vi "PSTR-Check If Repair Needed.vi"(0 "Data in":T2, 9 "CFTS-PSTR":T1) -> (8 "needs repair":bool)   [LabVIEW 2020]
uses:
  Typedefs/PSTR-Data.ctl
  Typedefs/PSTR-Model Fit.ctl
  Typedefs/PSTR-Fit Parameters.ctl
  Typedefs/PSTR-File Info.ctl
  <vilib>/Analysis/baseanly.llb/Mean (DBL).vi
  <vilib>/Analysis/NI_AALBase.lvlib
  <vilib>/Analysis/NI_AALPro.lvlib
panel:
  # "NF x NL x 2 x Npts"
  # "NF x NL x Npts"
  # "NF x NL"
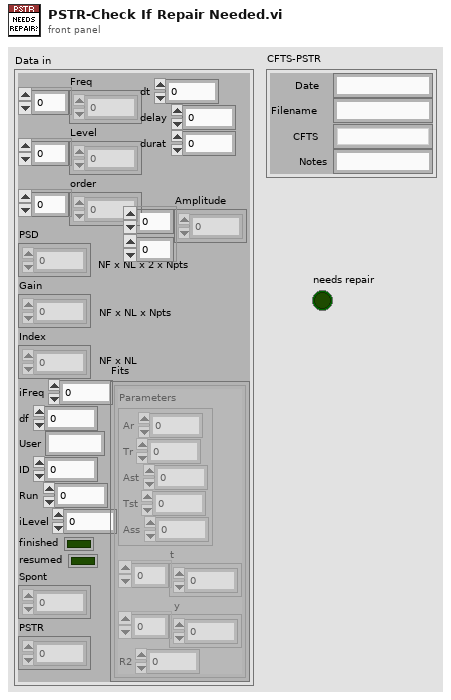
[diagram p1: front panel]
types:
  T1 = typedef "PSTR-File Info.ctl" = cluster{"Date":string, "Filename":string, "CFTS":string, "Notes":string}
  T2 = typedef "PSTR-Data.ctl" = cluster{"Freq":dbl[], "Level":dbl[], "order":i32[], "PSD":dbl[][][][], "Gain":dbl[][][], "Index":dbl[][], "iFreq":i32, "df":dbl, "User":string, "ID":i32, "Run":i32, "iLevel":i32, "finished":bool, "resumed":bool, "Spont":dbl[][], "PSTR":dbl[][][], "dt":dbl, "delay":dbl, "durat":dbl, "Fits":T3[][], "Amplitude":dbl[][]}
  T3 = typedef "PSTR-Model Fit.ctl" = cluster{"Parameters":T4, "t":dbl[], "y":dbl[], "R2":dbl}
  T4 = typedef "PSTR-Fit Parameters.ctl" = cluster{"Ar":dbl, "Tr":dbl, "Ast":dbl, "Tst":dbl, "Ass":dbl}
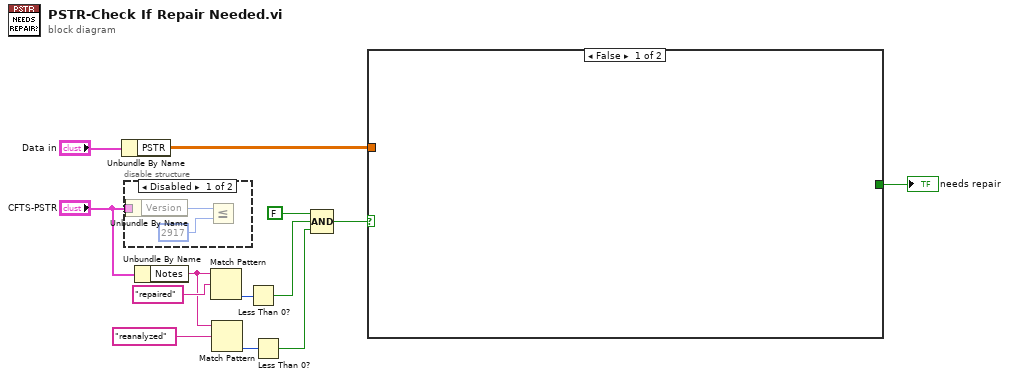
[diagram p0: block diagram]
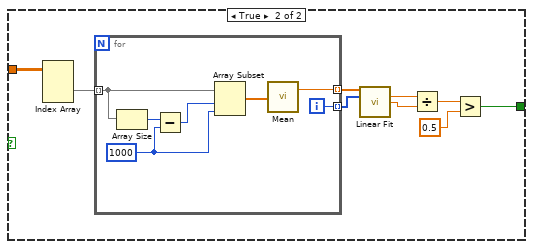
[diagram p3: hidden frame]
diagram:
  n1 = Unbundle By Name("Data in") -> ("PSTR"=w4:dbl[][][])
  n2 = disable-structure shown="Disabled" {
    disable-tunnel: "CFTS-PSTR" -> [w14 _]
    frame Disabled {
      n3 = Unbundle By Name(w14) -> ("Version"=w16:i32)
      n4 = Less Or Equal?(x=w16, y=2917) -> ()  [unwired: 1 out]
    }
    frame Enabled {
    }
  }
  n5 = Unbundle By Name("CFTS-PSTR") -> ("Notes"=w10:string)
  n6 = Match Pattern(string=w10, regular expression="repaired") -> (offset past match=w11:i32)  [unwired: 1 in, 3 out]
  n7 = Match Pattern(string=w10, regular expression="reanalyzed") -> (offset past match=w8:i32)  [unwired: 1 in, 3 out]
  n8 = Less Than 0?(x=w11) -> (x < 0?=w7:bool)
  n9 = Less Than 0?(x=w8) -> (x < 0?=w6:bool)
  n10 = Compound Arithmetic op=AND(FALSE ("value"), w7, w6) -> (w2:bool)
  n11 = case shown="False" w2 {
    tunnel: w4 -> [_ w25]
    tunnel: [_ w17] -> w3
    frame False {
    }
    frame True {
      n12 = Index Array(array=w25) -> (element=w24:dbl[][])  [unwired: 3 in]
      n13 = for {
        tunnel: w24 -> [w32] mode=indexing
        tunnel: [w27] -> w23 mode=indexing
        tunnel: [w26] -> w22 mode=indexing
        i -> [w26]
        w30 = 1000
        n14 = Array Size(array=w32) -> (size(s)=w31:i32)
        n15 = Subtract(x=w31, y=w30) -> (x-y=w29:i32)
        n16 = Array Subset(array=w32, index=w29, length=w30) -> (w28:dbl[])
        n17 = call-poly <vilib>:"Mean.vi"("X"=w28) -> ("mean"=w27:dbl)  [unwired: 1 out]
      }
      n18 = call <vilib>:"Linear Fit.vi"("Y"=w23, "X"=w22) -> ("slope"=w21:dbl, "intercept"=w20:dbl)  [unwired: 9 in, 3 out]
      n19 = Divide(x=w21, y=w20) -> (x/y=w19:dbl)
      n20 = Greater?(x=w19, y=0.5) -> (0:w17:bool)
    }
  }
  "needs repair" <- w3
